vi "Multi-camera acquisition of images.vi"() -> ()   [LabVIEW 2018]
uses:
  LabViewDVPCamera/LabViewDVPCamera.lvlib
  <vilib>/picture/picture.llb/imagedata.ctl
panel:
  out "Capture frame rate 4":sgl
  out "Total frame rate 4":u32
  out "pFrameCount out 4":T1
  out "Capture frame rate 3":sgl
  out "Total frame rate 3":u32
  out "pFrameCount out 3":T1
  out "Capture frame rate 2":sgl
  out "Total frame rate 2":u32
  out "pFrameCount out 2":T1
  out "Capture frame rate":sgl
  out "Total frame rate":u32
  out "pFrameCount out":T1
  out "frame rate 4":dbl format="%#.5g"
  out "number 4":u64
  out "new picture 4":picture caption="新图片"
  in  "CloseFlg 4":i32
  in  "CameraList 4":u16(ring) caption="CameraList" items=["MGS130M-192.168.0.251"]
  out "Set 4":bool
  out "Open 4":bool
  out "Close 4":bool
  out "ScanCamera 4":bool
  out "handle 4":u32
  in  "image data 4":T2 caption="图像数据"
  out "Millisecond timing value 6":u32
  out "frame rate 3":dbl format="%#.5g"
  out "number 3":u64
  out "new picture 3":picture caption="新图片"
  in  "CloseFlg 3":i32
  in  "CameraList 3":u16(ring) caption="CameraList" items=["MGS130M-192.168.0.251"]
  in  "Set 3":bool
  in  "Open 3":bool
  in  "Close 3":bool
  in  "ScanCamera 3":bool
  out "handle 3":u32
  in  "image data 3":T2 caption="图像数据"
  out "Millisecond timing value 5":u32
  out "frame rate 2":dbl format="%#.5g"
  out "number 2":u64
  out "new picture 2":picture caption="新图片"
  out "CloseFlg 2":i32
  in  "CameraList 2":u16(ring) caption="CameraList" items=["MGS130M-192.168.0.251"]
  out "Set 2":bool
  out "Open 2":bool
  out "Close 2":bool
  out "ScanCamera 2":bool
  out "handle 2":u32
  in  "image data 2":T2 caption="图像数据"
  out "Millisecond timing value 4":u32
  in  "image data":T2 caption="图像数据"
  out "Millisecond timing value 3":u32
  out "frame rate":dbl format="%#.5g"
  out "number":u64
  out "new picture":picture caption="新图片"
  in  "CloseFlg":i32
  in  "CameraList":u16(ring) items=["MGS130M-192.168.0.251"]
  in  "Set":bool
  in  "Open":bool
  out "Close":bool
  in  "ScanCamera":bool
  out "handle":u32
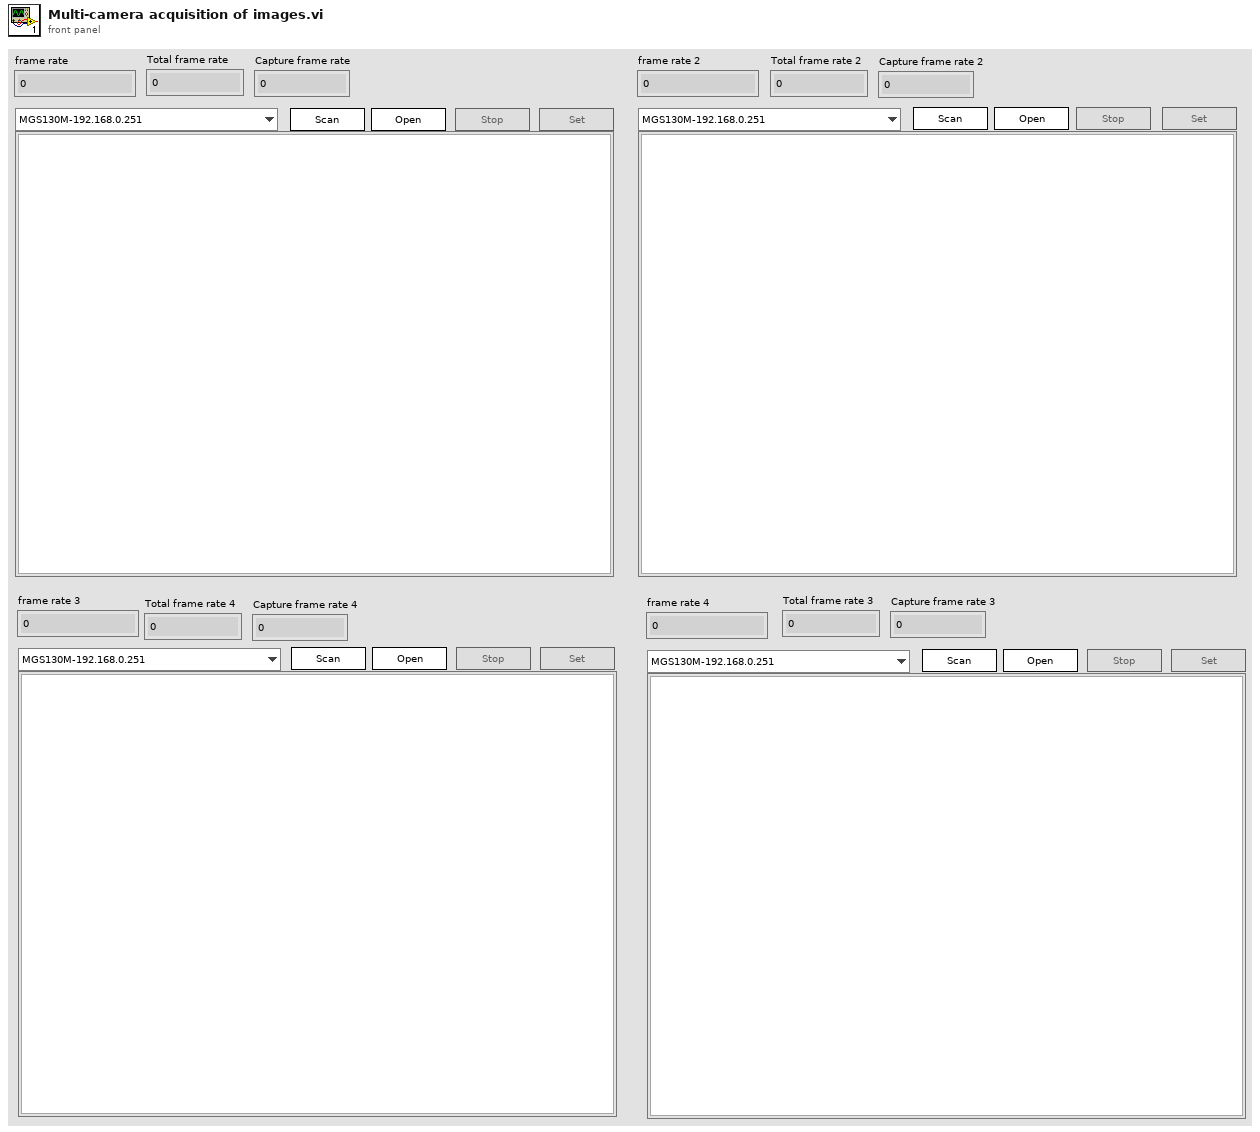
[diagram p1: front panel]
types:
  T1 = cluster{"uFrameCount":u32, "uFrameDrop":u32, "uFrameIgnore":u32, "uFrameError":u32, "uFrameOK":u32, "uFrameOut":u32, "uFrameResend":u32, "uFrameProc":u32, "fFrameRate":sgl, "fProcRate":sgl, "reserved[0]":i32, "reserved[1]":i32, "reserved[2]":i32, "reserved[3]":i32, "reserved[4]":i32, "reserved[5]":i32, "reserved[6]":i32, "reserved[7]":i32, "reserved[8]":i32, "reserved[9]":i32, "reserved[10]":i32, "reserved[11]":i32, "reserved[12]":i32, "reserved[13]":i32, "reserved[14]":i32, "reserved[15]":i32, "reserved[16]":i32, "reserved[17]":i32, "reserved[18]":i32, "reserved[19]":i32, "reserved[20]":i32, "reserved[21]":i32, "reserved[22]":i32, "reserved[23]":i32, "reserved[24]":i32, "reserved[25]":i32, "reserved[26]":i32, "reserved[27]":i32, "reserved[28]":i32, "reserved[29]":i32, "reserved[30]":i32, "reserved[31]":i32}
  T2 = typedef "imagedata.ctl" = cluster{"image type":i32, "image depth":i32, "image":u8[], "mask":u8[], "colors":u32[], "Rectangle":cluster{"left":i16, "top":i16, "right":i16, "bottom":i16}}
  T3 = enum8{"Enabled", "Disabled", "Disabled and Grayed Out"}
  T4 = typedef "LVStringsAndValuesArrayTypeDef_U16.ctl" = cluster{"String":string, "Value":u16}[]
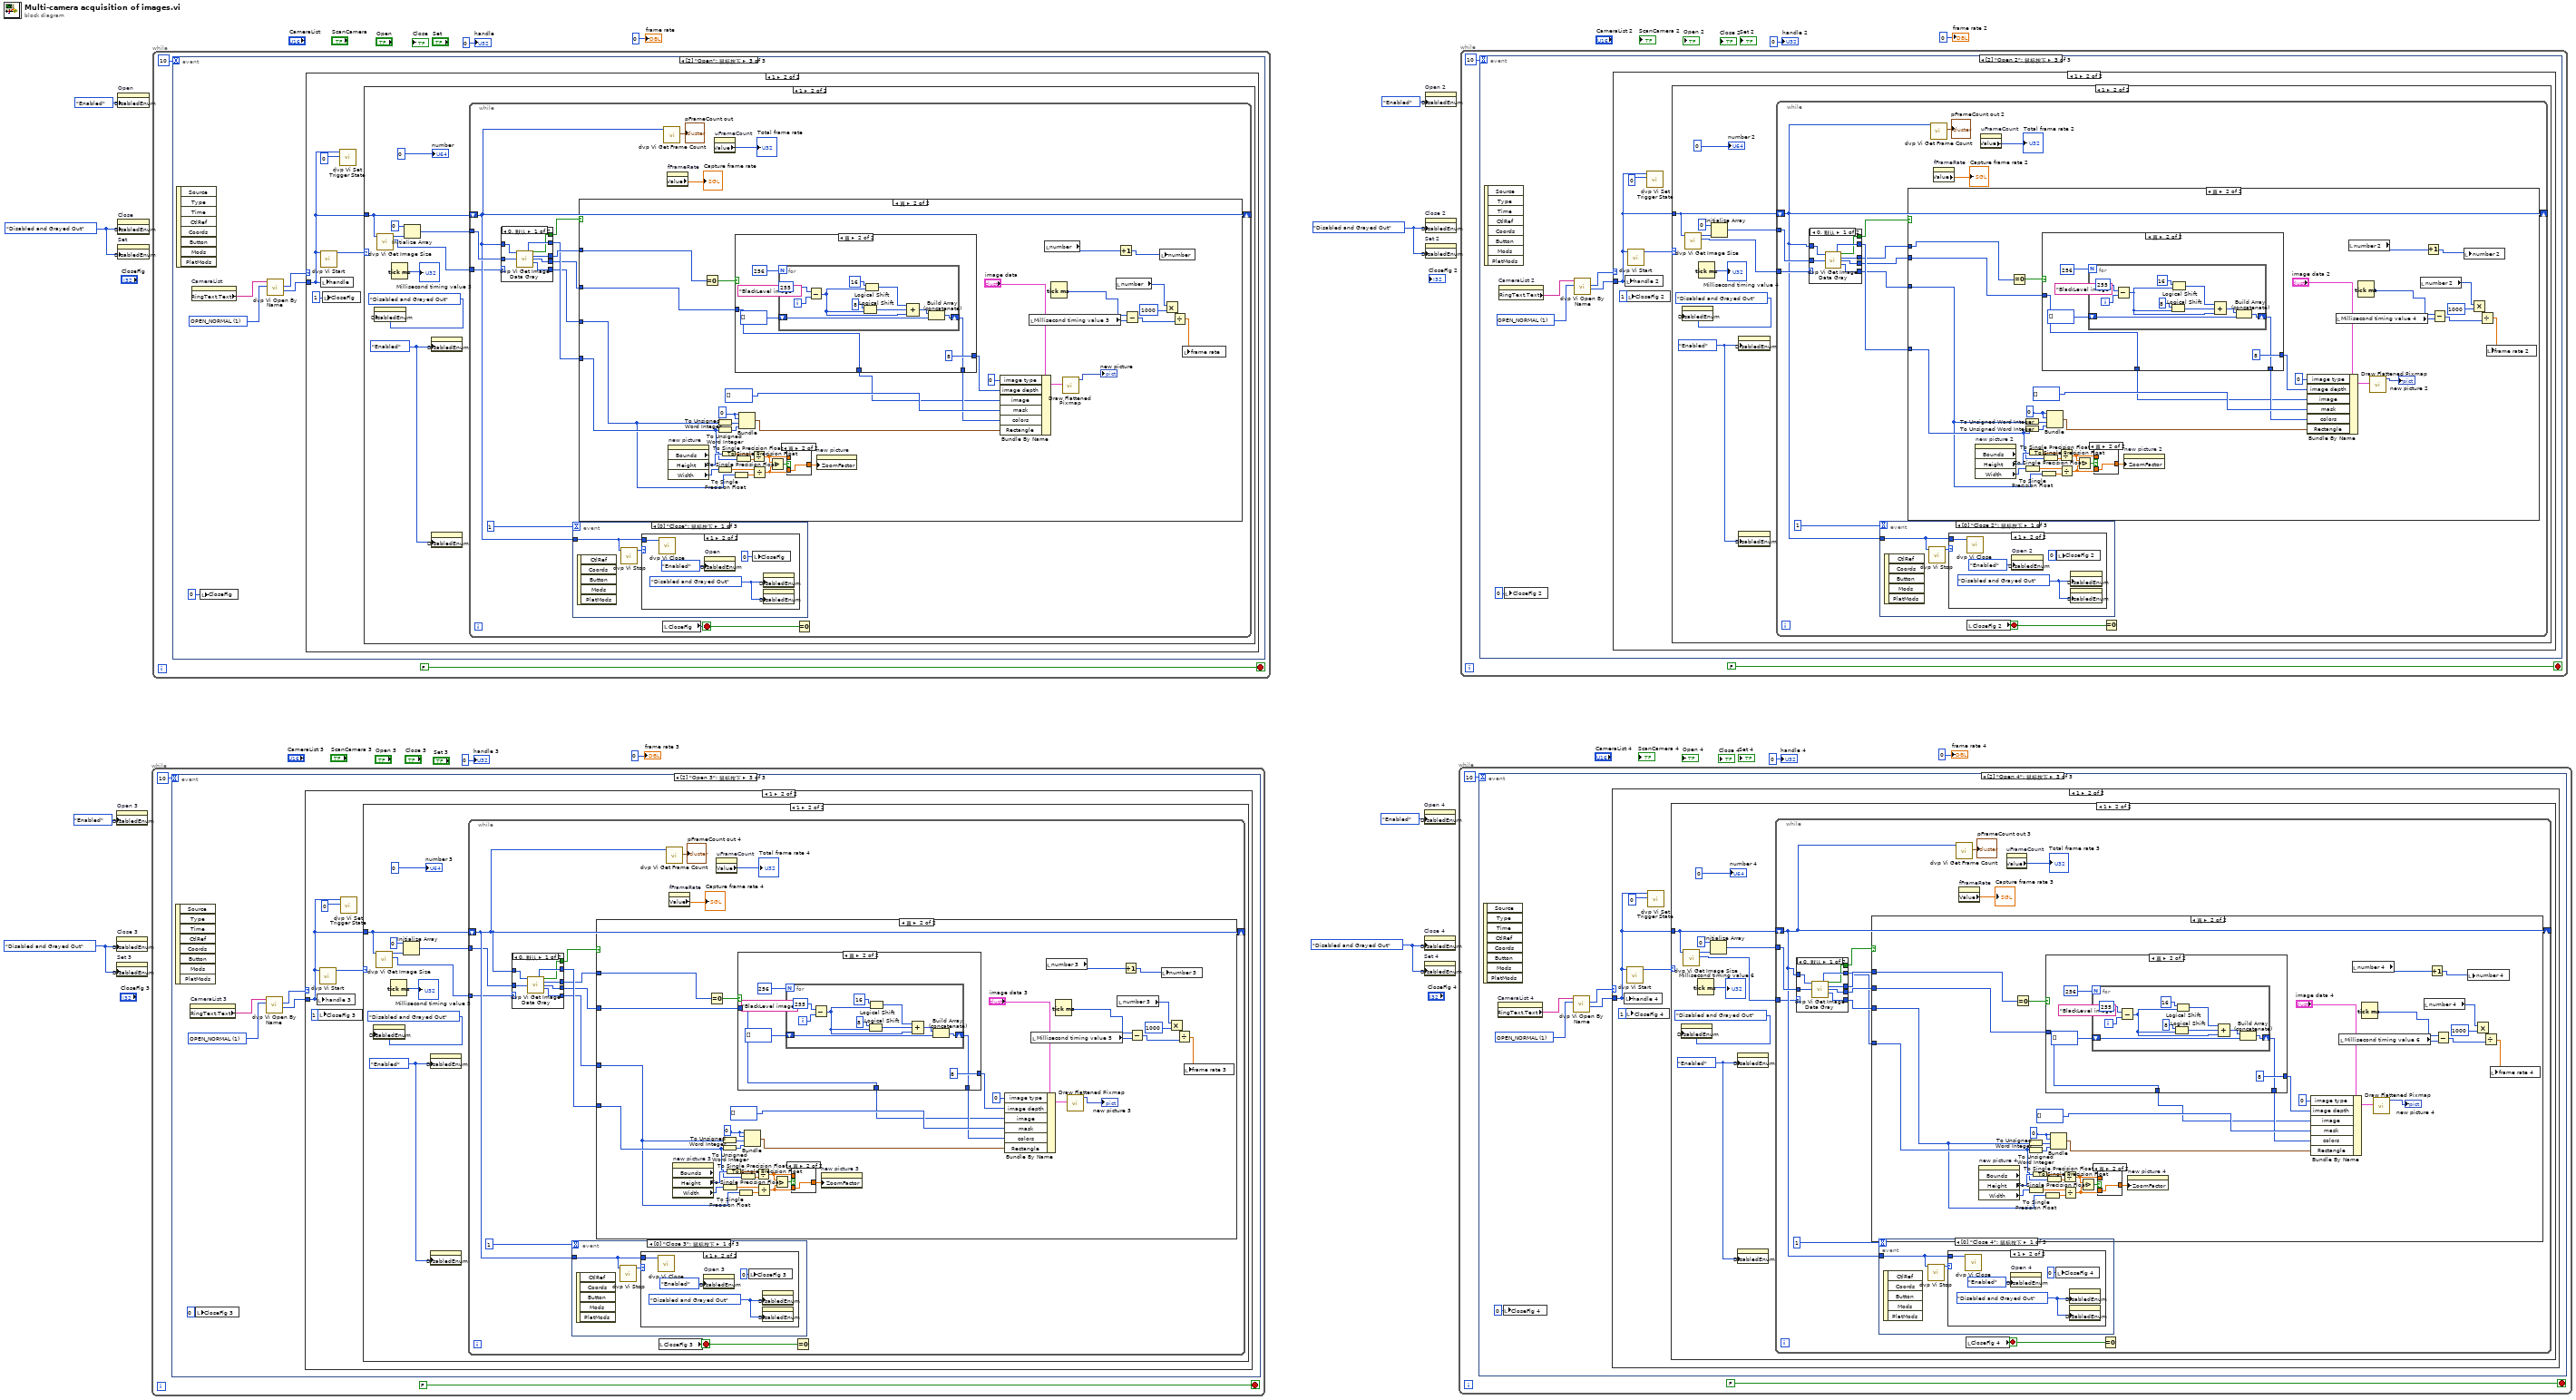
[diagram p0: block diagram]
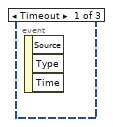
[diagram p2: hidden frame]
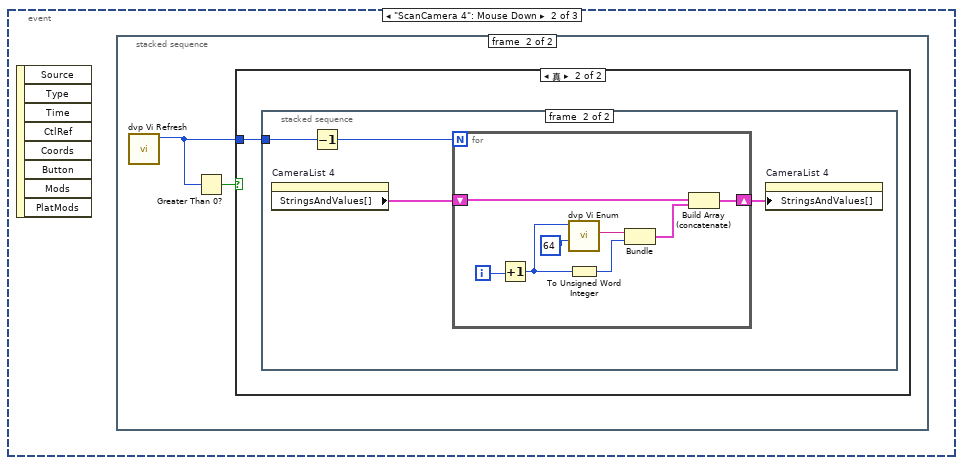
[diagram p3: hidden frame]
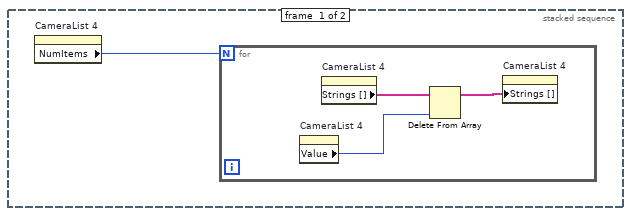
[diagram p4: hidden frame]
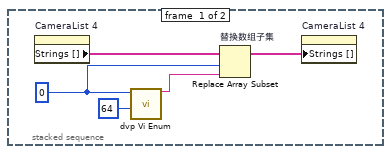
[diagram p6: hidden frame]
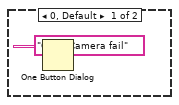
[diagram p7: hidden frame]
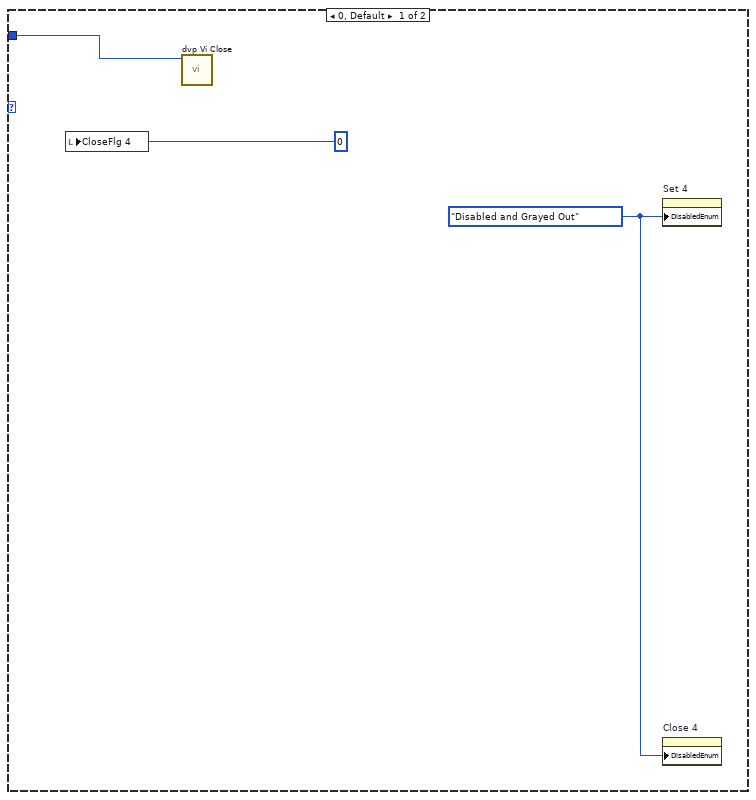
[diagram p8: hidden frame]
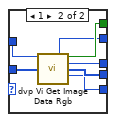
[diagram p9: hidden frame]
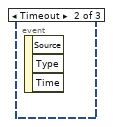
[diagram p11: hidden frame]
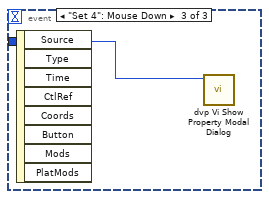
[diagram p12: hidden frame]
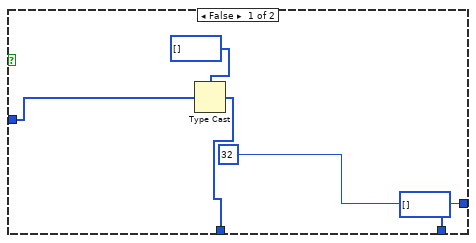
[diagram p15: hidden frame]
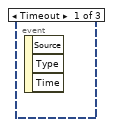
[diagram p16: hidden frame]
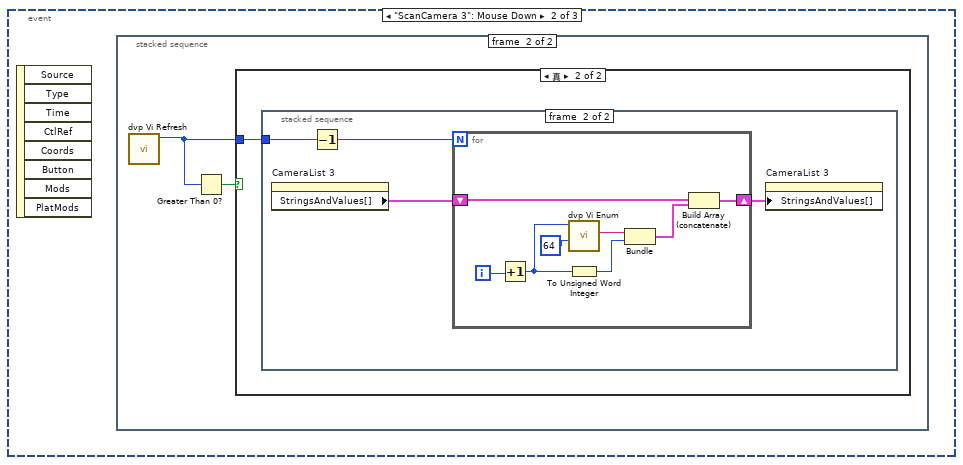
[diagram p17: hidden frame]
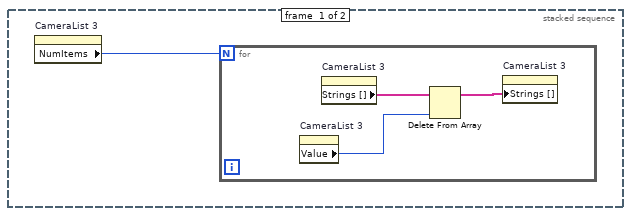
[diagram p18: hidden frame]
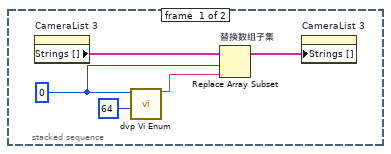
[diagram p20: hidden frame]
diagram:
  w3 = T3."Disabled and Grayed Out" ("禁用")
  w7 = T3."Disabled and Grayed Out" ("禁用")
  w11 = T3."Disabled and Grayed Out" ("禁用")
  w15 = T3."Disabled and Grayed Out" ("禁用")
  n1 = property on="Open 3" class="Bool"("DisabledEnum"=T3."Enabled" ("禁用")) -> ()  [unwired: 2 in, 2 out]
  n2 = property on="Close 3" class="Bool"("DisabledEnum"=w7) -> ()  [unwired: 2 in, 2 out]
  n3 = property on="Set 3" class="Bool"("DisabledEnum"=w7) -> ()  [unwired: 2 in, 2 out]
  n4 = property on="Open" class="Bool"("DisabledEnum"=T3."Enabled" ("禁用")) -> ()  [unwired: 2 in, 2 out]
  n5 = property on="Close" class="Bool"("DisabledEnum"=w15) -> ()  [unwired: 2 in, 2 out]
  n6 = property on="Set" class="Bool"("DisabledEnum"=w15) -> ()  [unwired: 2 in, 2 out]
  n7 = while {
    stop <- FALSE stop-if-true
    n8 = event shown="[2] \"Open 3\": 鼠标按下" {
      selector: _ -> [_ _ _]
      dyn-events: _ -> [_ _ _]
      timeout: 10 -> [_ _ _]
      event Timeout {
        n9 = event-data() -> ()  [unwired: 1 in, 3 out]
      }
      event "ScanCamera 3": Mouse Down {
        n10 = event-data() -> ()  [unwired: 1 in, 8 out]
        n11 = stacked-sequence "清除下拉列表的数据" {
          frame #0 {
            n12 = property on="CameraList 3" class="Ring (严格)"() -> ("NumItems"=w19:u32)  [unwired: 2 in, 2 out]
            n13 = for {
              N: w19 -> [_]
              n14 = property on="CameraList 3" class="Ring (严格)"() -> ("Value"=w21:u16)  [unwired: 2 in, 2 out]
              n15 = property on="CameraList 3" class="Ring (严格)"() -> ("Strings []"=w20:string[])  [unwired: 2 in, 2 out]
              n16 = Delete From Array ("删除数组元素")(array=w20, index=w21) -> (array with subset deleted=w22:string[])  [unwired: 1 in, 1 out]
              n17 = property on="CameraList 3" class="Ring (严格)"("Strings []"=w22) -> ()  [unwired: 2 in, 2 out]
            }
          }
          frame #1 {
            n18 = call "dvp Vi Refresh.vi"() -> ("pCount out"=w24:u32)  [unwired: 10 in, 1 out]
            n19 = Greater Than 0?(x=w24) -> (x > 0?=w23:bool)
            n20 = case shown="真" w23 {
              tunnel: w24 -> [_ w25]
              frame False {
              }
              frame True {
                n21 = stacked-sequence {
                  tunnel: w25 -> [_ w32]
                  frame #0 {
                    w26 = u32 0 ("index")
                    n22 = property on="CameraList 3" class="Ring (严格)"() -> ("Strings []"=w29:string[])  [unwired: 2 in, 2 out]
                    n23 = call "dvp Vi Enum.vi"("unSize"=u32 64, "index"=w26) -> ("friendlyName out"=w28:string)  [unwired: 8 in, 1 out]
                    n24 = Replace Array Subset "替换数组子集"(array=w29, new element=w28, index=w26) -> (w30:string[])
                    n25 = property on="CameraList 3" class="Ring (严格)"("Strings []"=w30) -> ()  [unwired: 2 in, 2 out]
                  }
                  frame #1 {
                    n26 = property on="CameraList 3" class="Ring (严格)"() -> ("StringsAndValues[]"=w34:T4)  [unwired: 2 in, 2 out]
                    n27 = Decrement(x=w32) -> (x-1=w31:u32)
                    n28 = for {
                      N: w31 -> [_]
                      shift-right: [w41] -> w33
                      shift-left: w34 -> [w39]
                      i -> [w36]
                      n29 = Increment(x=w36) -> (x+1=w35:i32)
                      n30 = call "dvp Vi Enum.vi"("unSize"=u32 64, "index"=w35) -> ("friendlyName out"=w42:string)  [unwired: 8 in, 1 out]
                      n31 = To Unsigned Word Integer(number=w35) -> (unsigned 16bit integer=w38:u16)
                      n32 = Bundle("friendlyName out"=w42, w38) -> (w40:cluster{"friendlyName out":string, u16})  [unwired: 1 in]
                      n33 = Build Array (concatenate)(w39, w40) -> (w41:T4)
                    }
                    n34 = property on="CameraList 3" class="Ring (严格)"("StringsAndValues[]"=w33) -> ()  [unwired: 2 in, 2 out]
                  }
                }
              }
            }
          }
        }
      }
      event "Open 3": Mouse Down {
        w45 = u32 1 items=["OPEN_OFFLINE", "OPEN_NORMAL"] ("type")
        n35 = event-data() -> ()  [unwired: 1 in, 8 out]
        n36 = property on="CameraList 3" class="Ring (严格)"() -> ("RingText.Text"=w44:string)  [unwired: 2 in, 2 out]
        n37 = local write "CloseFlg 3"(0 ("CloseFlg")) -> ()
        n38 = call "dvp Vi Open By Name.vi"("type"=w45, "friendlyName"=w44) -> ("pHandle out"=w47:u32, "function return"=w46:u32)  [unwired: 7 in, 1 out]
        n39 = case shown="1" w46 {
          tunnel: w47 -> [_ w49]
          frame 0, Default {
            n40 = One Button Dialog(message="Open Camera fail" ("消息")) -> ()  [unwired: 1 in, 1 out]
          }
          frame 1 {
            n41 = local write "handle 3"(w49) -> ()
            n42 = local write "CloseFlg 3"(1 ("CloseFlg")) -> ()
            n43 = call "dvp Vi Start.vi"("handle"=w49) -> ("function return"=w51:u32)  [unwired: 10 in]
            n44 = call "dvp Vi Set Trigger State.vi"("TriggerState"=0, "handle"=w49) -> ()  [unwired: 9 in, 1 out]
            n45 = case shown="1" w51 {
              tunnel: w49 -> [w55 w60]
              frame 0, Default {
                w54 = T3."Disabled and Grayed Out" ("禁用")
                n46 = local write "CloseFlg 3"(0 ("CloseFlg")) -> ()
                n47 = call "dvp Vi Close.vi"("handle"=w55) -> ()  [unwired: 10 in, 1 out]
                n48 = property on="Set 3" class="Bool"("DisabledEnum"=w54) -> ()  [unwired: 2 in, 2 out]
                n49 = property on="Close 3" class="Bool"("DisabledEnum"=w54) -> ()  [unwired: 2 in, 2 out]
              }
              frame 1 {
                w64 = T3."Enabled" ("禁用")
                n50 = property on="Open 3" class="Bool"("DisabledEnum"=T3."Disabled and Grayed Out" ("禁用")) -> ()  [unwired: 2 in, 2 out]
                n51 = call "dvp Vi Get Image Size.vi"("handle"=w60) -> ("pformat out"=w57:i32, "function return"=w59:u32)  [unwired: 9 in]
                n52 = Tick Count (ms)() -> (millisecond timer value=→"Millisecond timing value 5":u32)
                n53 = Initialize Array(u32 0 ("元素"), w59) -> (w61:u32[])
                n54 = property on="Set 3" class="Bool"("DisabledEnum"=w64) -> ()  [unwired: 2 in, 2 out]
                n55 = property on="Close 3" class="Bool"("DisabledEnum"=w64) -> ()  [unwired: 2 in, 2 out]
                n56 = while {
                  shift-right: [w72] -> _
                  shift-left: w60 -> [w72]
                  tunnel: w61 -> [w71]
                  tunnel: w57 -> [w70]
                  stop <- w77 stop-if-true
                  n57 = case shown="0, 默认" w70 {
                    tunnel: w71 -> [w85 w92]
                    tunnel: w72 -> [w84 w91]
                    tunnel: [w80 w90] -> w69
                    tunnel: [w82 w89] -> w66
                    tunnel: [w81 w88] -> w67
                    tunnel: [w83 w87] -> w68
                    tunnel: [w79 w86] -> w65
                    frame 0, Default {
                      n58 = call "dvp Vi Get Image Data Gray.vi"("handle"=w84, "pbuffer"=w85) -> ("piHeight out"=w83:i32, "function return"=w80:bool, "pformat out"=w81:i32, "pbuffer out"=w82:u8[], "piWidth out"=w79:i32)  [unwired: 9 in]
                    }
                    frame 1 {
                      n59 = call "dvp Vi Get Image Data Rgb.vi"("handle"=w91, "pbuffer"=w92) -> ("piHeight out"=w87:i32, "function return"=w90:bool, "pformat out"=w88:i32, "pbuffer out"=w89:u32[], "piWidth out"=w86:i32)  [unwired: 9 in]
                    }
                  }
                  n60 = event shown="[0] \"Close 3\": 鼠标按下" {
                    selector: _ -> [_ _ _]
                    dyn-events: _ -> [_ _ _]
                    timeout: 1 -> [_ _ _]
                    tunnel: w72 -> [w93 _ w99]
                    event "Close 3": Mouse Down {
                      n61 = event-data() -> ()  [unwired: 1 in, 5 out]
                      n62 = call "dvp Vi Stop.vi"("handle"=w93) -> ("function return"=w94:u32)  [unwired: 10 in]
                      n63 = case shown="1" w94 {
                        tunnel: w93 -> [_ w96]
                        frame 0, Default {
                        }
                        frame 1 {
                          w95 = T3."Disabled and Grayed Out" ("禁用")
                          n64 = call "dvp Vi Close.vi"("handle"=w96) -> ()  [unwired: 10 in, 1 out]
                          n65 = property on="Open 3" class="Bool"("DisabledEnum"=T3."Enabled" ("禁用")) -> ()  [unwired: 2 in, 2 out]
                          n66 = local write "CloseFlg 3"(0 ("CloseFlg")) -> ()
                          n67 = property on="Close 3" class="Bool"("DisabledEnum"=w95) -> ()  [unwired: 2 in, 2 out]
                          n68 = property on="Set 3" class="Bool"("DisabledEnum"=w95) -> ()  [unwired: 2 in, 2 out]
                        }
                      }
                    }
                    event Timeout {
                      n69 = event-data() -> ()  [unwired: 1 in, 3 out]
                    }
                    event "Set 3": Mouse Down {
                      n70 = event-data() -> ()  [unwired: 1 in, 8 out]
                      n71 = call "dvp Vi Show Property Modal Dialog.vi"("handle"=w99) -> ()  [unwired: 10 in, 1 out]
                    }
                  }
                  n72 = case shown="真" w69 {
                    tunnel: w66 -> [_ w102]
                    tunnel: w65 -> [_ w104]
                    tunnel: w68 -> [_ w105]
                    tunnel: w67 -> [_ w106]
                    frame False {
                    }
                    frame True {
                      w135 = u16 0
                      n73 = property on="new picture 3" class="Pict" props=["Bounds", "Height", "Width"]() -> ("Height"=w107:u32, "Width"=w108:u32)  [unwired: 2 in, 3 out]
                      n74 = Equal To 0?(x=w106) -> (x = 0?=w132:bool)
                      n75 = To Unsigned Word Integer(number=w104) -> (unsigned 16bit integer=w134:u16)
                      n76 = To Unsigned Word Integer(number=w105) -> (unsigned 16bit integer=w133:u16)
                      n77 = To Single Precision Float(number=w108) -> (single precision float=w115:sgl)
                      n78 = To Single Precision Float(number=w107) -> (single precision float=w109:sgl)
                      n79 = case shown="真" w132 {
                        tunnel: [32 u8 8 ("image depth")] -> w129
                        tunnel: [i32[] [] ("数组") w144] -> w127
                        tunnel: w102 -> [w139 w143]
                        tunnel: [w138 w143] -> w101
                        frame False {
                          n80 = Type Cast(type=u8[] [], x=w139) -> (*(type *) &x=w138:u8[])
                        }
                        frame True {
                          (unwired) "BlackLevel image"
                          n81 = for {
                            N: 256 -> [_]
                            shift-right: [w152] -> w144
                            shift-left: i32[] [] ("数组") -> [w151]
                            i -> [w148]
                            n82 = Subtract(x=255, y=w148) -> (x-y=w149:i32)
                            n83 = Logical Shift(y=i16 8, x=w149) -> (x << y=w154:i32)
                            n84 = Logical Shift(y=16 ("x"), x=w149) -> (x << y=w155:i32)
                            n85 = Compound Arithmetic op=ADD(w155, w154, w149) -> (w153:i32)
                            n86 = Build Array (concatenate)(w153, w151) -> (w152:i32[])
                          }
                        }
                      }
                      n87 = To Single Precision Float(number=w104) -> (single precision float=w111:sgl)
                      n88 = To Single Precision Float(number=w105) -> (single precision float=w110:sgl)
                      n89 = Bundle ("图像尺寸")(w135, w135, w134, w133) -> (w126:cluster{u16, u16, u16, u16})  [unwired: 1 in]
                      n90 = Divide(x=w109, y=w110) -> (x/y=w113:sgl)
                      n91 = Divide(x=w115, y=w111) -> (x/y=w114:sgl)
                      n92 = Greater?(x=w113, y=w114) -> (0:w112:bool)
                      n93 = case shown="真" w112 {
                        tunnel: w113 -> [w136 _]
                        tunnel: w114 -> [_ w137]
                        tunnel: [w136 w137] -> w116
                        frame False {
                        }
                        frame True {
                        }
                      }
                      n94 = property on="new picture 3" class="Pict"("ZoomFactor"=w116) -> ()  [unwired: 2 in, 2 out]
                      n95 = Bundle By Name(cluster="image data 3", "image type"=0, "image depth"=w129, "image"=w101, "mask"=u8[] [] ("无符号8位数组"), "colors"=w127, "Rectangle"=w126) -> (w130:T2)
                      n96 = local read "Millisecond timing value 5"() -> (w103:u32)
                      n97 = local read "number 3"() -> (w121:u64)
                      n98 = Tick Count (ms)() -> (millisecond timer value=w119:u32)
                      n99 = call <vilib>:"Draw Flattened Pixmap.vi"("image data"=w130) -> ("new picture"=→"new picture 3":picture)  [unwired: 8 in]
                      n100 = local read "number 3"() -> (w118:u64)
                      n101 = Increment(x=w121) -> (x+1=w120:u64)
                      n102 = Subtract(x=w119, y=w103) -> (x-y=w124:u32)
                      n103 = local write "number 3"(w120) -> ()
                      n104 = Multiply(x=w118, y=u64 1000) -> (x*y=w122:u64)
                      n105 = Divide(x=w122, y=w124) -> (x/y=w117:dbl)
                      n106 = local write "frame rate 3"(w117) -> ()
                    }
                  }
                  n107 = local read "CloseFlg 3"() -> (w76:i32)
                  n108 = call "dvp Vi Get Frame Count.vi"("handle"=w72) -> ("pFrameCount out"=→"pFrameCount out 4":T1)  [unwired: 9 in, 1 out]
                  n109 = property on="fFrameRate" class="DigNum (严格)"() -> ("Value"=→"Capture frame rate 4":sgl)  [unwired: 2 in, 2 out]
                  n110 = property on="uFrameCount" class="DigNum (严格)"() -> ("Value"=→"Total frame rate 4":u32)  [unwired: 2 in, 2 out]
                  n111 = Equal To 0?(x=w76) -> (x = 0?=w77:bool)
                }
                "number 3" <- u64 0
              }
            }
          }
        }
      }
    }
  }
  n112 = while {
    stop <- FALSE stop-if-true
    n113 = event shown="[2] \"Open\": 鼠标按下" {
      selector: _ -> [_ _ _]
      dyn-events: _ -> [_ _ _]
      timeout: 10 -> [_ _ _]
      event Timeout {
        n114 = event-data() -> ()  [unwired: 1 in, 3 out]
      }
      event "ScanCamera": Mouse Down {
        n115 = event-data() -> ()  [unwired: 1 in, 8 out]
        n116 = stacked-sequence "清除下拉列表的数据" {
          frame #0 {
            n117 = property on="CameraList" class="Ring (严格)"() -> ("NumItems"=w160:u32)  [unwired: 2 in, 2 out]
            n118 = for {
              N: w160 -> [_]
              n119 = property on="CameraList" class="Ring (严格)"() -> ("Value"=w162:u16)  [unwired: 2 in, 2 out]
              n120 = property on="CameraList" class="Ring (严格)"() -> ("Strings []"=w161:string[])  [unwired: 2 in, 2 out]
              n121 = Delete From Array ("删除数组元素")(array=w161, index=w162) -> (array with subset deleted=w163:string[])  [unwired: 1 in, 1 out]
              n122 = property on="CameraList" class="Ring (严格)"("Strings []"=w163) -> ()  [unwired: 2 in, 2 out]
            }
          }
          frame #1 {
            n123 = call "dvp Vi Refresh.vi"() -> ("pCount out"=w165:u32)  [unwired: 10 in, 1 out]
            n124 = Greater Than 0?(x=w165) -> (x > 0?=w164:bool)
            n125 = case shown="真" w164 {
              tunnel: w165 -> [_ w166]
              frame False {
              }
              frame True {
                n126 = stacked-sequence {
                  tunnel: w166 -> [_ w173]
                  frame #0 {
                    w167 = u32 0 ("index")
                    n127 = property on="CameraList" class="Ring (严格)"() -> ("Strings []"=w170:string[])  [unwired: 2 in, 2 out]
                    n128 = call "dvp Vi Enum.vi"("unSize"=u32 64, "index"=w167) -> ("friendlyName out"=w169:string)  [unwired: 8 in, 1 out]
                    n129 = Replace Array Subset "替换数组子集"(array=w170, new element=w169, index=w167) -> (w171:string[])
                    n130 = property on="CameraList" class="Ring (严格)"("Strings []"=w171) -> ()  [unwired: 2 in, 2 out]
                  }
                  frame #1 {
                    n131 = property on="CameraList" class="Ring (严格)"() -> ("StringsAndValues[]"=w175:T4)  [unwired: 2 in, 2 out]
                    n132 = Decrement(x=w173) -> (x-1=w172:u32)
                    n133 = for {
                      N: w172 -> [_]
                      shift-right: [w182] -> w174
                      shift-left: w175 -> [w180]
                      i -> [w177]
                      n134 = Increment(x=w177) -> (x+1=w176:i32)
                      n135 = call "dvp Vi Enum.vi"("unSize"=u32 64, "index"=w176) -> ("friendlyName out"=w183:string)  [unwired: 8 in, 1 out]
                      n136 = To Unsigned Word Integer(number=w176) -> (unsigned 16bit integer=w179:u16)
                      n137 = Bundle("friendlyName out"=w183, w179) -> (w181:cluster{"friendlyName out":string, u16})  [unwired: 1 in]
                      n138 = Build Array (concatenate)(w180, w181) -> (w182:T4)
                    }
                    n139 = property on="CameraList" class="Ring (严格)"("StringsAndValues[]"=w174) -> ()  [unwired: 2 in, 2 out]
                  }
                }
              }
            }
          }
        }
      }
      event "Open": Mouse Down {
        w186 = u32 1 items=["OPEN_OFFLINE", "OPEN_NORMAL"] ("type")
        n140 = event-data() -> ()  [unwired: 1 in, 8 out]
        n141 = property on="CameraList" class="Ring (严格)"() -> ("RingText.Text"=w185:string)  [unwired: 2 in, 2 out]
        n142 = local write "CloseFlg"(0 ("CloseFlg")) -> ()
        n143 = call "dvp Vi Open By Name.vi"("type"=w186, "friendlyName"=w185) -> ("pHandle out"=w188:u32, "function return"=w187:u32)  [unwired: 7 in, 1 out]
        n144 = case shown="1" w187 {
          tunnel: w188 -> [_ w190]
          frame 0, Default {
            n145 = One Button Dialog(message="Open Camera fail" ("消息")) -> ()  [unwired: 1 in, 1 out]
          }
          frame 1 {
            n146 = call "dvp Vi Start.vi"("handle"=w190) -> ("function return"=w192:u32)  [unwired: 10 in]
            n147 = local write "handle"(w190) -> ()
            n148 = local write "CloseFlg"(1 ("CloseFlg")) -> ()
            n149 = call "dvp Vi Set Trigger State.vi"("TriggerState"=0, "handle"=w190) -> ()  [unwired: 9 in, 1 out]
            n150 = case shown="1" w192 {
              tunnel: w190 -> [w196 w201]
              frame 0, Default {
                w195 = T3."Disabled and Grayed Out" ("禁用")
                n151 = local write "CloseFlg"(0 ("CloseFlg")) -> ()
                n152 = call "dvp Vi Close.vi"("handle"=w196) -> ()  [unwired: 10 in, 1 out]
                n153 = property on="Set" class="Bool"("DisabledEnum"=w195) -> ()  [unwired: 2 in, 2 out]
                n154 = property on="Close" class="Bool"("DisabledEnum"=w195) -> ()  [unwired: 2 in, 2 out]
              }
              frame 1 {
                w205 = T3."Enabled" ("禁用")
                n155 = property on="Open" class="Bool"("DisabledEnum"=T3."Disabled and Grayed Out" ("禁用")) -> ()  [unwired: 2 in, 2 out]
                n156 = call "dvp Vi Get Image Size.vi"("handle"=w201) -> ("pformat out"=w198:i32, "function return"=w200:u32)  [unwired: 9 in]
                n157 = Tick Count (ms)() -> (millisecond timer value=→"Millisecond timing value 3":u32)
                n158 = Initialize Array(u32 0 ("元素"), w200) -> (w202:u32[])
                n159 = property on="Set" class="Bool"("DisabledEnum"=w205) -> ()  [unwired: 2 in, 2 out]
                n160 = property on="Close" class="Bool"("DisabledEnum"=w205) -> ()  [unwired: 2 in, 2 out]
                n161 = while {
                  shift-right: [w207] -> _
                  shift-left: w201 -> [w207]
                  tunnel: w202 -> [w208]
                  tunnel: w198 -> [w206]
                  stop <- w218 stop-if-true
                  n162 = case shown="0, 默认" w206 {
                    tunnel: w208 -> [w226 w233]
                    tunnel: w207 -> [w225 w232]
                    tunnel: [w221 w231] -> w213
                    tunnel: [w223 w230] -> w209
                    tunnel: [w222 w229] -> w212
                    tunnel: [w224 w228] -> w211
                    tunnel: [w220 w227] -> w210
                    frame 0, Default {
                      n163 = call "dvp Vi Get Image Data Gray.vi"("handle"=w225, "pbuffer"=w226) -> ("piHeight out"=w224:i32, "function return"=w221:bool, "pformat out"=w222:i32, "pbuffer out"=w223:u8[], "piWidth out"=w220:i32)  [unwired: 9 in]
                    }
                    frame 1 {
                      n164 = call "dvp Vi Get Image Data Rgb.vi"("handle"=w232, "pbuffer"=w233) -> ("piHeight out"=w228:i32, "function return"=w231:bool, "pformat out"=w229:i32, "pbuffer out"=w230:u32[], "piWidth out"=w227:i32)  [unwired: 9 in]
                    }
                  }
                  n165 = event shown="[0] \"Close\": 鼠标按下" {
                    selector: _ -> [_ _ _]
                    dyn-events: _ -> [_ _ _]
                    timeout: 1 -> [_ _ _]
                    tunnel: w207 -> [w234 _ w240]
                    event "Close": Mouse Down {
                      n166 = event-data() -> ()  [unwired: 1 in, 5 out]
                      n167 = call "dvp Vi Stop.vi"("handle"=w234) -> ("function return"=w235:u32)  [unwired: 10 in]
                      n168 = case shown="1" w235 {
                        tunnel: w234 -> [_ w237]
                        frame 0, Default {
                        }
                        frame 1 {
                          w236 = T3."Disabled and Grayed Out" ("禁用")
                          n169 = call "dvp Vi Close.vi"("handle"=w237) -> ()  [unwired: 10 in, 1 out]
                          n170 = property on="Open" class="Bool"("DisabledEnum"=T3."Enabled" ("禁用")) -> ()  [unwired: 2 in, 2 out]
                          n171 = local write "CloseFlg"(0 ("CloseFlg")) -> ()
                          n172 = property on="Close" class="Bool"("DisabledEnum"=w236) -> ()  [unwired: 2 in, 2 out]
                          n173 = property on="Set" class="Bool"("DisabledEnum"=w236) -> ()  [unwired: 2 in, 2 out]
                        }
                      }
                    }
                    event Timeout {
                      n174 = event-data() -> ()  [unwired: 1 in, 3 out]
                    }
                    event "Set": Mouse Down {
                      n175 = event-data() -> ()  [unwired: 1 in, 8 out]
                      n176 = call "dvp Vi Show Property Modal Dialog.vi"("handle"=w240) -> ()  [unwired: 10 in, 1 out]
                    }
                  }
                  n177 = case shown="真" w213 {
                    tunnel: w209 -> [_ w243]
                    tunnel: w210 -> [_ w245]
                    tunnel: w211 -> [_ w246]
                    tunnel: w212 -> [_ w247]
                    frame False {
                    }
                    frame True {
                      w276 = u16 0
                      n178 = property on="new picture" class="Pict" props=["Bounds", "Height", "Width"]() -> ("Height"=w248:u32, "Width"=w249:u32)  [unwired: 2 in, 3 out]
                      n179 = Equal To 0?(x=w247) -> (x = 0?=w273:bool)
                      n180 = To Unsigned Word Integer(number=w245) -> (unsigned 16bit integer=w275:u16)
                      n181 = To Unsigned Word Integer(number=w246) -> (unsigned 16bit integer=w274:u16)
                      n182 = To Single Precision Float(number=w249) -> (single precision float=w256:sgl)
                      n183 = To Single Precision Float(number=w248) -> (single precision float=w250:sgl)
                      n184 = To Single Precision Float(number=w245) -> (single precision float=w252:sgl)
                      n185 = case shown="真" w273 {
                        tunnel: [32 u8 8 ("image depth")] -> w270
                        tunnel: [i32[] [] ("数组") w285] -> w268
                        tunnel: w243 -> [w280 w284]
                        tunnel: [w279 w284] -> w242
                        frame False {
                          n186 = Type Cast(type=u8[] [], x=w280) -> (*(type *) &x=w279:u8[])
                        }
                        frame True {
                          (unwired) "BlackLevel image"
                          n187 = for {
                            N: 256 -> [_]
                            shift-right: [w293] -> w285
                            shift-left: i32[] [] ("数组") -> [w292]
                            i -> [w289]
                            n188 = Subtract(x=255, y=w289) -> (x-y=w290:i32)
                            n189 = Logical Shift(y=i16 8, x=w290) -> (x << y=w295:i32)
                            n190 = Logical Shift(y=16 ("x"), x=w290) -> (x << y=w296:i32)
                            n191 = Compound Arithmetic op=ADD(w296, w295, w290) -> (w294:i32)
                            n192 = Build Array (concatenate)(w294, w292) -> (w293:i32[])
                          }
                        }
                      }
                      n193 = To Single Precision Float(number=w246) -> (single precision float=w251:sgl)
                      n194 = Bundle ("图像尺寸")(w276, w276, w275, w274) -> (w267:cluster{u16, u16, u16, u16})  [unwired: 1 in]
                      n195 = Divide(x=w250, y=w251) -> (x/y=w254:sgl)
                      n196 = Divide(x=w256, y=w252) -> (x/y=w255:sgl)
                      n197 = Greater?(x=w254, y=w255) -> (0:w253:bool)
                      n198 = case shown="真" w253 {
                        tunnel: w254 -> [w277 _]
                        tunnel: w255 -> [_ w278]
                        tunnel: [w277 w278] -> w257
                        frame False {
                        }
                        frame True {
                        }
                      }
                      n199 = property on="new picture" class="Pict"("ZoomFactor"=w257) -> ()  [unwired: 2 in, 2 out]
                      n200 = Bundle By Name(cluster="image data", "image type"=0, "image depth"=w270, "image"=w242, "mask"=u8[] [] ("无符号8位数组"), "colors"=w268, "Rectangle"=w267) -> (w271:T2)
                      n201 = local read "Millisecond timing value 3"() -> (w244:u32)
                      n202 = local read "number"() -> (w262:u64)
                      n203 = Tick Count (ms)() -> (millisecond timer value=w260:u32)
                      n204 = call <vilib>:"Draw Flattened Pixmap.vi"("image data"=w271) -> ("new picture"=→"new picture":picture)  [unwired: 8 in]
                      n205 = local read "number"() -> (w259:u64)
                      n206 = Increment(x=w262) -> (x+1=w261:u64)
                      n207 = Subtract(x=w260, y=w244) -> (x-y=w265:u32)
                      n208 = local write "number"(w261) -> ()
                      n209 = Multiply(x=w259, y=u64 1000) -> (x*y=w263:u64)
                      n210 = Divide(x=w263, y=w265) -> (x/y=w258:dbl)
                      n211 = local write "frame rate"(w258) -> ()
                    }
                  }
                  n212 = local read "CloseFlg"() -> (w217:i32)
                  n213 = call "dvp Vi Get Frame Count.vi"("handle"=w207) -> ("pFrameCount out"=→"pFrameCount out":T1)  [unwired: 9 in, 1 out]
                  n214 = property on="fFrameRate" class="DigNum (严格)"() -> ("Value"=→"Capture frame rate":sgl)  [unwired: 2 in, 2 out]
                  n215 = property on="uFrameCount" class="DigNum (严格)"() -> ("Value"=→"Total frame rate":u32)  [unwired: 2 in, 2 out]
                  n216 = Equal To 0?(x=w217) -> (x = 0?=w218:bool)
                }
                "number" <- u64 0
              }
            }
          }
        }
      }
    }
  }
  n217 = property on="Open 4" class="Bool"("DisabledEnum"=T3."Enabled" ("禁用")) -> ()  [unwired: 2 in, 2 out]
  n218 = property on="Close 4" class="Bool"("DisabledEnum"=w3) -> ()  [unwired: 2 in, 2 out]
  n219 = property on="Set 4" class="Bool"("DisabledEnum"=w3) -> ()  [unwired: 2 in, 2 out]
  n220 = property on="Open 2" class="Bool"("DisabledEnum"=T3."Enabled" ("禁用")) -> ()  [unwired: 2 in, 2 out]
  n221 = property on="Close 2" class="Bool"("DisabledEnum"=w11) -> ()  [unwired: 2 in, 2 out]
  n222 = property on="Set 2" class="Bool"("DisabledEnum"=w11) -> ()  [unwired: 2 in, 2 out]
  n223 = while {
    stop <- FALSE stop-if-true
    n224 = event shown="[2] \"Open 4\": 鼠标按下" {
      selector: _ -> [_ _ _]
      dyn-events: _ -> [_ _ _]
      timeout: 10 -> [_ _ _]
      event Timeout {
        n225 = event-data() -> ()  [unwired: 1 in, 3 out]
      }
      event "ScanCamera 4": Mouse Down {
        n226 = event-data() -> ()  [unwired: 1 in, 8 out]
        n227 = stacked-sequence "清除下拉列表的数据" {
          frame #0 {
            n228 = property on="CameraList 4" class="Ring (严格)"() -> ("NumItems"=w301:u32)  [unwired: 2 in, 2 out]
            n229 = for {
              N: w301 -> [_]
              n230 = property on="CameraList 4" class="Ring (严格)"() -> ("Value"=w303:u16)  [unwired: 2 in, 2 out]
              n231 = property on="CameraList 4" class="Ring (严格)"() -> ("Strings []"=w302:string[])  [unwired: 2 in, 2 out]
              n232 = Delete From Array ("删除数组元素")(array=w302, index=w303) -> (array with subset deleted=w304:string[])  [unwired: 1 in, 1 out]
              n233 = property on="CameraList 4" class="Ring (严格)"("Strings []"=w304) -> ()  [unwired: 2 in, 2 out]
            }
          }
          frame #1 {
            n234 = call "dvp Vi Refresh.vi"() -> ("pCount out"=w306:u32)  [unwired: 10 in, 1 out]
            n235 = Greater Than 0?(x=w306) -> (x > 0?=w305:bool)
            n236 = case shown="真" w305 {
              tunnel: w306 -> [_ w307]
              frame False {
              }
              frame True {
                n237 = stacked-sequence {
                  tunnel: w307 -> [_ w314]
                  frame #0 {
                    w308 = u32 0 ("index")
                    n238 = property on="CameraList 4" class="Ring (严格)"() -> ("Strings []"=w311:string[])  [unwired: 2 in, 2 out]
                    n239 = call "dvp Vi Enum.vi"("unSize"=u32 64, "index"=w308) -> ("friendlyName out"=w310:string)  [unwired: 8 in, 1 out]
                    n240 = Replace Array Subset "替换数组子集"(array=w311, new element=w310, index=w308) -> (w312:string[])
                    n241 = property on="CameraList 4" class="Ring (严格)"("Strings []"=w312) -> ()  [unwired: 2 in, 2 out]
                  }
                  frame #1 {
                    n242 = property on="CameraList 4" class="Ring (严格)"() -> ("StringsAndValues[]"=w316:T4)  [unwired: 2 in, 2 out]
                    n243 = Decrement(x=w314) -> (x-1=w313:u32)
                    n244 = for {
                      N: w313 -> [_]
                      shift-right: [w323] -> w315
                      shift-left: w316 -> [w321]
                      i -> [w318]
                      n245 = Increment(x=w318) -> (x+1=w317:i32)
                      n246 = call "dvp Vi Enum.vi"("unSize"=u32 64, "index"=w317) -> ("friendlyName out"=w324:string)  [unwired: 8 in, 1 out]
                      n247 = To Unsigned Word Integer(number=w317) -> (unsigned 16bit integer=w320:u16)
                      n248 = Bundle("friendlyName out"=w324, w320) -> (w322:cluster{"friendlyName out":string, u16})  [unwired: 1 in]
                      n249 = Build Array (concatenate)(w321, w322) -> (w323:T4)
                    }
                    n250 = property on="CameraList 4" class="Ring (严格)"("StringsAndValues[]"=w315) -> ()  [unwired: 2 in, 2 out]
                  }
                }
              }
            }
          }
        }
      }
      event "Open 4": Mouse Down {
        w327 = u32 1 items=["OPEN_OFFLINE", "OPEN_NORMAL"] ("type")
        n251 = event-data() -> ()  [unwired: 1 in, 8 out]
        n252 = property on="CameraList 4" class="Ring (严格)"() -> ("RingText.Text"=w326:string)  [unwired: 2 in, 2 out]
        n253 = local write "CloseFlg 4"(0 ("CloseFlg")) -> ()
        n254 = call "dvp Vi Open By Name.vi"("type"=w327, "friendlyName"=w326) -> ("pHandle out"=w329:u32, "function return"=w328:u32)  [unwired: 7 in, 1 out]
        n255 = case shown="1" w328 {
          tunnel: w329 -> [_ w331]
          frame 0, Default {
            n256 = One Button Dialog(message="Open Camera fail" ("消息")) -> ()  [unwired: 1 in, 1 out]
          }
          frame 1 {
            n257 = local write "handle 4"(w331) -> ()
            n258 = local write "CloseFlg 4"(1 ("CloseFlg")) -> ()
            n259 = call "dvp Vi Start.vi"("handle"=w331) -> ("function return"=w333:u32)  [unwired: 10 in]
            n260 = call "dvp Vi Set Trigger State.vi"("TriggerState"=0, "handle"=w331) -> ()  [unwired: 9 in, 1 out]
            n261 = case shown="1" w333 {
              tunnel: w331 -> [w337 w342]
              frame 0, Default {
                w336 = T3."Disabled and Grayed Out" ("禁用")
                n262 = local write "CloseFlg 4"(0 ("CloseFlg")) -> ()
                n263 = call "dvp Vi Close.vi"("handle"=w337) -> ()  [unwired: 10 in, 1 out]
                n264 = property on="Set 4" class="Bool"("DisabledEnum"=w336) -> ()  [unwired: 2 in, 2 out]
                n265 = property on="Close 4" class="Bool"("DisabledEnum"=w336) -> ()  [unwired: 2 in, 2 out]
              }
              frame 1 {
                w346 = T3."Enabled" ("禁用")
                n266 = property on="Open 4" class="Bool"("DisabledEnum"=T3."Disabled and Grayed Out" ("禁用")) -> ()  [unwired: 2 in, 2 out]
                n267 = call "dvp Vi Get Image Size.vi"("handle"=w342) -> ("pformat out"=w339:i32, "function return"=w341:u32)  [unwired: 9 in]
                n268 = Tick Count (ms)() -> (millisecond timer value=→"Millisecond timing value 6":u32)
                n269 = Initialize Array(u32 0 ("元素"), w341) -> (w343:u32[])
                n270 = property on="Set 4" class="Bool"("DisabledEnum"=w346) -> ()  [unwired: 2 in, 2 out]
                n271 = property on="Close 4" class="Bool"("DisabledEnum"=w346) -> ()  [unwired: 2 in, 2 out]
                n272 = while {
                  shift-right: [w353] -> _
                  shift-left: w342 -> [w353]
                  tunnel: w343 -> [w354]
                  tunnel: w339 -> [w352]
                  stop <- w359 stop-if-true
                  n273 = case shown="0, 默认" w352 {
                    tunnel: w354 -> [w367 w374]
                    tunnel: w353 -> [w366 w373]
                    tunnel: [w362 w372] -> w349
                    tunnel: [w364 w371] -> w351
                    tunnel: [w363 w370] -> w350
                    tunnel: [w365 w369] -> w347
                    tunnel: [w361 w368] -> w348
                    frame 0, Default {
                      n274 = call "dvp Vi Get Image Data Gray.vi"("handle"=w366, "pbuffer"=w367) -> ("piHeight out"=w365:i32, "function return"=w362:bool, "pformat out"=w363:i32, "pbuffer out"=w364:u8[], "piWidth out"=w361:i32)  [unwired: 9 in]
                    }
                    frame 1 {
                      n275 = call "dvp Vi Get Image Data Rgb.vi"("handle"=w373, "pbuffer"=w374) -> ("piHeight out"=w369:i32, "function return"=w372:bool, "pformat out"=w370:i32, "pbuffer out"=w371:u32[], "piWidth out"=w368:i32)  [unwired: 9 in]
                    }
                  }
                  n276 = case shown="真" w349 {
                    tunnel: w351 -> [_ w383]
                    tunnel: w348 -> [_ w386]
                    tunnel: w347 -> [_ w387]
                    tunnel: w350 -> [_ w388]
                    frame False {
                    }
                    frame True {
                      w417 = u16 0
                      n277 = property on="new picture 4" class="Pict" props=["Bounds", "Height", "Width"]() -> ("Height"=w389:u32, "Width"=w390:u32)  [unwired: 2 in, 3 out]
                      n278 = Equal To 0?(x=w388) -> (x = 0?=w414:bool)
                      n279 = To Unsigned Word Integer(number=w386) -> (unsigned 16bit integer=w416:u16)
                      n280 = To Unsigned Word Integer(number=w387) -> (unsigned 16bit integer=w415:u16)
                      n281 = To Single Precision Float(number=w390) -> (single precision float=w397:sgl)
                      n282 = To Single Precision Float(number=w389) -> (single precision float=w391:sgl)
                      n283 = To Single Precision Float(number=w386) -> (single precision float=w393:sgl)
                      n284 = case shown="真" w414 {
                        tunnel: [32 u8 8 ("image depth")] -> w411
                        tunnel: [i32[] [] ("数组") w426] -> w409
                        tunnel: [w421 w425] -> w384
                        tunnel: w383 -> [w420 w425]
                        frame False {
                          n285 = Type Cast(type=u8[] [], x=w420) -> (*(type *) &x=w421:u8[])
                        }
                        frame True {
                          (unwired) "BlackLevel image"
                          n286 = for {
                            N: 256 -> [_]
                            shift-right: [w434] -> w426
                            shift-left: i32[] [] ("数组") -> [w433]
                            i -> [w430]
                            n287 = Subtract(x=255, y=w430) -> (x-y=w431:i32)
                            n288 = Logical Shift(y=i16 8, x=w431) -> (x << y=w436:i32)
                            n289 = Logical Shift(y=16 ("x"), x=w431) -> (x << y=w437:i32)
                            n290 = Compound Arithmetic op=ADD(w437, w436, w431) -> (w435:i32)
                            n291 = Build Array (concatenate)(w435, w433) -> (w434:i32[])
                          }
                        }
                      }
                      n292 = To Single Precision Float(number=w387) -> (single precision float=w392:sgl)
                      n293 = Bundle ("图像尺寸")(w417, w417, w416, w415) -> (w408:cluster{u16, u16, u16, u16})  [unwired: 1 in]
                      n294 = Divide(x=w391, y=w392) -> (x/y=w395:sgl)
                      n295 = Divide(x=w397, y=w393) -> (x/y=w396:sgl)
                      n296 = Greater?(x=w395, y=w396) -> (0:w394:bool)
                      n297 = case shown="真" w394 {
                        tunnel: w395 -> [w418 _]
                        tunnel: w396 -> [_ w419]
                        tunnel: [w418 w419] -> w398
                        frame False {
                        }
                        frame True {
                        }
                      }
                      n298 = property on="new picture 4" class="Pict"("ZoomFactor"=w398) -> ()  [unwired: 2 in, 2 out]
                      n299 = Bundle By Name(cluster="image data 4", "image type"=0, "image depth"=w411, "image"=w384, "mask"=u8[] [] ("无符号8位数组"), "colors"=w409, "Rectangle"=w408) -> (w412:T2)
                      n300 = local read "Millisecond timing value 6"() -> (w385:u32)
                      n301 = local read "number 4"() -> (w403:u64)
                      n302 = Tick Count (ms)() -> (millisecond timer value=w401:u32)
                      n303 = call <vilib>:"Draw Flattened Pixmap.vi"("image data"=w412) -> ("new picture"=→"new picture 4":picture)  [unwired: 8 in]
                      n304 = local read "number 4"() -> (w400:u64)
                      n305 = Increment(x=w403) -> (x+1=w402:u64)
                      n306 = Subtract(x=w401, y=w385) -> (x-y=w406:u32)
                      n307 = local write "number 4"(w402) -> ()
                      n308 = Multiply(x=w400, y=u64 1000) -> (x*y=w404:u64)
                      n309 = Divide(x=w404, y=w406) -> (x/y=w399:dbl)
                      n310 = local write "frame rate 4"(w399) -> ()
                    }
                  }
                  n311 = event shown="[0] \"Close 4\": 鼠标按下" {
                    selector: _ -> [_ _ _]
                    dyn-events: _ -> [_ _ _]
                    timeout: 1 -> [_ _ _]
                    tunnel: w353 -> [w375 _ w381]
                    event "Close 4": Mouse Down {
                      n312 = event-data() -> ()  [unwired: 1 in, 5 out]
                      n313 = call "dvp Vi Stop.vi"("handle"=w375) -> ("function return"=w376:u32)  [unwired: 10 in]
                      n314 = case shown="1" w376 {
                        tunnel: w375 -> [_ w378]
                        frame 0, Default {
                        }
                        frame 1 {
                          w377 = T3."Disabled and Grayed Out" ("禁用")
                          n315 = call "dvp Vi Close.vi"("handle"=w378) -> ()  [unwired: 10 in, 1 out]
                          n316 = property on="Open 4" class="Bool"("DisabledEnum"=T3."Enabled" ("禁用")) -> ()  [unwired: 2 in, 2 out]
                          n317 = local write "CloseFlg 4"(0 ("CloseFlg")) -> ()
                          n318 = property on="Close 4" class="Bool"("DisabledEnum"=w377) -> ()  [unwired: 2 in, 2 out]
                          n319 = property on="Set 4" class="Bool"("DisabledEnum"=w377) -> ()  [unwired: 2 in, 2 out]
                        }
                      }
                    }
                    event Timeout {
                      n320 = event-data() -> ()  [unwired: 1 in, 3 out]
                    }
                    event "Set 4": Mouse Down {
                      n321 = event-data() -> ()  [unwired: 1 in, 8 out]
                      n322 = call "dvp Vi Show Property Modal Dialog.vi"("handle"=w381) -> ()  [unwired: 10 in, 1 out]
                    }
                  }
                  n323 = call "dvp Vi Get Frame Count.vi"("handle"=w353) -> ("pFrameCount out"=→"pFrameCount out 3":T1)  [unwired: 9 in, 1 out]
                  n324 = property on="fFrameRate" class="DigNum (严格)"() -> ("Value"=→"Capture frame rate 3":sgl)  [unwired: 2 in, 2 out]
                  n325 = local read "CloseFlg 4"() -> (w358:i32)
                  n326 = property on="uFrameCount" class="DigNum (严格)"() -> ("Value"=→"Total frame rate 3":u32)  [unwired: 2 in, 2 out]
                  n327 = Equal To 0?(x=w358) -> (x = 0?=w359:bool)
                }
                "number 4" <- u64 0
              }
            }
          }
        }
      }
    }
  }
  n328 = while {
    stop <- FALSE stop-if-true
    n329 = event shown="[2] \"Open 2\": 鼠标按下" {
      selector: _ -> [_ _ _]
      dyn-events: _ -> [_ _ _]
      timeout: 10 -> [_ _ _]
      event Timeout {
        n330 = event-data() -> ()  [unwired: 1 in, 3 out]
      }
      event "ScanCamera 2": Mouse Down {
        n331 = event-data() -> ()  [unwired: 1 in, 8 out]
        n332 = stacked-sequence "清除下拉列表的数据" {
          frame #0 {
            n333 = property on="CameraList 2" class="Ring (严格)"() -> ("NumItems"=w442:u32)  [unwired: 2 in, 2 out]
            n334 = for {
              N: w442 -> [_]
              n335 = property on="CameraList 2" class="Ring (严格)"() -> ("Value"=w444:u16)  [unwired: 2 in, 2 out]
              n336 = property on="CameraList 2" class="Ring (严格)"() -> ("Strings []"=w443:string[])  [unwired: 2 in, 2 out]
              n337 = Delete From Array ("删除数组元素")(array=w443, index=w444) -> (array with subset deleted=w445:string[])  [unwired: 1 in, 1 out]
              n338 = property on="CameraList 2" class="Ring (严格)"("Strings []"=w445) -> ()  [unwired: 2 in, 2 out]
            }
          }
          frame #1 {
            n339 = call "dvp Vi Refresh.vi"() -> ("pCount out"=w447:u32)  [unwired: 10 in, 1 out]
            n340 = Greater Than 0?(x=w447) -> (x > 0?=w446:bool)
            n341 = case shown="真" w446 {
              tunnel: w447 -> [_ w448]
              frame False {
              }
              frame True {
                n342 = stacked-sequence {
                  tunnel: w448 -> [_ w455]
                  frame #0 {
                    w449 = u32 0 ("index")
                    n343 = property on="CameraList 2" class="Ring (严格)"() -> ("Strings []"=w452:string[])  [unwired: 2 in, 2 out]
                    n344 = call "dvp Vi Enum.vi"("unSize"=u32 64, "index"=w449) -> ("friendlyName out"=w451:string)  [unwired: 8 in, 1 out]
                    n345 = Replace Array Subset "替换数组子集"(array=w452, new element=w451, index=w449) -> (w453:string[])
                    n346 = property on="CameraList 2" class="Ring (严格)"("Strings []"=w453) -> ()  [unwired: 2 in, 2 out]
                  }
                  frame #1 {
                    n347 = property on="CameraList 2" class="Ring (严格)"() -> ("StringsAndValues[]"=w457:T4)  [unwired: 2 in, 2 out]
                    n348 = Decrement(x=w455) -> (x-1=w454:u32)
                    n349 = for {
                      N: w454 -> [_]
                      shift-right: [w464] -> w456
                      shift-left: w457 -> [w462]
                      i -> [w459]
                      n350 = Increment(x=w459) -> (x+1=w458:i32)
                      n351 = call "dvp Vi Enum.vi"("unSize"=u32 64, "index"=w458) -> ("friendlyName out"=w465:string)  [unwired: 8 in, 1 out]
                      n352 = To Unsigned Word Integer(number=w458) -> (unsigned 16bit integer=w461:u16)
                      n353 = Bundle("friendlyName out"=w465, w461) -> (w463:cluster{"friendlyName out":string, u16})  [unwired: 1 in]
                      n354 = Build Array (concatenate)(w462, w463) -> (w464:T4)
                    }
                    n355 = property on="CameraList 2" class="Ring (严格)"("StringsAndValues[]"=w456) -> ()  [unwired: 2 in, 2 out]
                  }
                }
              }
            }
          }
        }
      }
      event "Open 2": Mouse Down {
        w468 = u32 1 items=["OPEN_OFFLINE", "OPEN_NORMAL"] ("type")
        n356 = event-data() -> ()  [unwired: 1 in, 8 out]
        n357 = property on="CameraList 2" class="Ring (严格)"() -> ("RingText.Text"=w467:string)  [unwired: 2 in, 2 out]
        n358 = local write "CloseFlg 2"(0 ("CloseFlg")) -> ()
        n359 = call "dvp Vi Open By Name.vi"("type"=w468, "friendlyName"=w467) -> ("pHandle out"=w470:u32, "function return"=w469:u32)  [unwired: 7 in, 1 out]
        n360 = case shown="1" w469 {
          tunnel: w470 -> [_ w472]
          frame 0, Default {
            n361 = One Button Dialog(message="Open Camera fail" ("消息")) -> ()  [unwired: 1 in, 1 out]
          }
          frame 1 {
            n362 = local write "handle 2"(w472) -> ()
            n363 = local write "CloseFlg 2"(1 ("CloseFlg")) -> ()
            n364 = call "dvp Vi Start.vi"("handle"=w472) -> ("function return"=w474:u32)  [unwired: 10 in]
            n365 = call "dvp Vi Set Trigger State.vi"("TriggerState"=0, "handle"=w472) -> ()  [unwired: 9 in, 1 out]
            n366 = case shown="1" w474 {
              tunnel: w472 -> [w478 w483]
              frame 0, Default {
                w477 = T3."Disabled and Grayed Out" ("禁用")
                n367 = local write "CloseFlg 2"(0 ("CloseFlg")) -> ()
                n368 = call "dvp Vi Close.vi"("handle"=w478) -> ()  [unwired: 10 in, 1 out]
                n369 = property on="Set 2" class="Bool"("DisabledEnum"=w477) -> ()  [unwired: 2 in, 2 out]
                n370 = property on="Close 2" class="Bool"("DisabledEnum"=w477) -> ()  [unwired: 2 in, 2 out]
              }
              frame 1 {
                w487 = T3."Enabled" ("禁用")
                n371 = property on="Open 2" class="Bool"("DisabledEnum"=T3."Disabled and Grayed Out" ("禁用")) -> ()  [unwired: 2 in, 2 out]
                n372 = call "dvp Vi Get Image Size.vi"("handle"=w483) -> ("pformat out"=w480:i32, "function return"=w482:u32)  [unwired: 9 in]
                n373 = Tick Count (ms)() -> (millisecond timer value=→"Millisecond timing value 4":u32)
                n374 = Initialize Array(u32 0 ("元素"), w482) -> (w484:u32[])
                n375 = property on="Set 2" class="Bool"("DisabledEnum"=w487) -> ()  [unwired: 2 in, 2 out]
                n376 = property on="Close 2" class="Bool"("DisabledEnum"=w487) -> ()  [unwired: 2 in, 2 out]
                n377 = while {
                  shift-right: [w488] -> _
                  shift-left: w483 -> [w488]
                  tunnel: w484 -> [w489]
                  tunnel: w480 -> [w495]
                  stop <- w500 stop-if-true
                  n378 = case shown="0, 默认" w495 {
                    tunnel: w489 -> [w508 w515]
                    tunnel: w488 -> [w507 w514]
                    tunnel: [w503 w513] -> w494
                    tunnel: [w505 w512] -> w491
                    tunnel: [w504 w511] -> w492
                    tunnel: [w506 w510] -> w493
                    tunnel: [w502 w509] -> w490
                    frame 0, Default {
                      n379 = call "dvp Vi Get Image Data Gray.vi"("handle"=w507, "pbuffer"=w508) -> ("piHeight out"=w506:i32, "function return"=w503:bool, "pformat out"=w504:i32, "pbuffer out"=w505:u8[], "piWidth out"=w502:i32)  [unwired: 9 in]
                    }
                    frame 1 {
                      n380 = call "dvp Vi Get Image Data Rgb.vi"("handle"=w514, "pbuffer"=w515) -> ("piHeight out"=w510:i32, "function return"=w513:bool, "pformat out"=w511:i32, "pbuffer out"=w512:u32[], "piWidth out"=w509:i32)  [unwired: 9 in]
                    }
                  }
                  n381 = event shown="[0] \"Close 2\": 鼠标按下" {
                    selector: _ -> [_ _ _]
                    dyn-events: _ -> [_ _ _]
                    timeout: 1 -> [_ _ _]
                    tunnel: w488 -> [w516 _ w522]
                    event "Close 2": Mouse Down {
                      n382 = event-data() -> ()  [unwired: 1 in, 5 out]
                      n383 = call "dvp Vi Stop.vi"("handle"=w516) -> ("function return"=w517:u32)  [unwired: 10 in]
                      n384 = case shown="1" w517 {
                        tunnel: w516 -> [_ w519]
                        frame 0, Default {
                        }
                        frame 1 {
                          w518 = T3."Disabled and Grayed Out" ("禁用")
                          n385 = call "dvp Vi Close.vi"("handle"=w519) -> ()  [unwired: 10 in, 1 out]
                          n386 = property on="Open 2" class="Bool"("DisabledEnum"=T3."Enabled" ("禁用")) -> ()  [unwired: 2 in, 2 out]
                          n387 = local write "CloseFlg 2"(0 ("CloseFlg")) -> ()
                          n388 = property on="Close 2" class="Bool"("DisabledEnum"=w518) -> ()  [unwired: 2 in, 2 out]
                          n389 = property on="Set 2" class="Bool"("DisabledEnum"=w518) -> ()  [unwired: 2 in, 2 out]
                        }
                      }
                    }
                    event Timeout {
                      n390 = event-data() -> ()  [unwired: 1 in, 3 out]
                    }
                    event "Set 2": Mouse Down {
                      n391 = event-data() -> ()  [unwired: 1 in, 8 out]
                      n392 = call "dvp Vi Show Property Modal Dialog.vi"("handle"=w522) -> ()  [unwired: 10 in, 1 out]
                    }
                  }
                  n393 = case shown="真" w494 {
                    tunnel: w491 -> [_ w525]
                    tunnel: w490 -> [_ w528]
                    tunnel: w493 -> [_ w529]
                    tunnel: w492 -> [_ w526]
                    frame False {
                    }
                    frame True {
                      w558 = u16 0
                      n394 = property on="new picture 2" class="Pict" props=["Bounds", "Height", "Width"]() -> ("Height"=w530:u32, "Width"=w531:u32)  [unwired: 2 in, 3 out]
                      n395 = Equal To 0?(x=w526) -> (x = 0?=w555:bool)
                      n396 = To Unsigned Word Integer(number=w528) -> (unsigned 16bit integer=w557:u16)
                      n397 = To Unsigned Word Integer(number=w529) -> (unsigned 16bit integer=w556:u16)
                      n398 = To Single Precision Float(number=w531) -> (single precision float=w538:sgl)
                      n399 = To Single Precision Float(number=w530) -> (single precision float=w532:sgl)
                      n400 = To Single Precision Float(number=w528) -> (single precision float=w534:sgl)
                      n401 = case shown="真" w555 {
                        tunnel: [32 u8 8 ("image depth")] -> w552
                        tunnel: [i32[] [] ("数组") w567] -> w550
                        tunnel: w525 -> [w562 w566]
                        tunnel: [w561 w566] -> w524
                        frame False {
                          n402 = Type Cast(type=u8[] [], x=w562) -> (*(type *) &x=w561:u8[])
                        }
                        frame True {
                          (unwired) "BlackLevel image"
                          n403 = for {
                            N: 256 -> [_]
                            shift-right: [w575] -> w567
                            shift-left: i32[] [] ("数组") -> [w574]
                            i -> [w571]
                            n404 = Subtract(x=255, y=w571) -> (x-y=w572:i32)
                            n405 = Logical Shift(y=i16 8, x=w572) -> (x << y=w577:i32)
                            n406 = Logical Shift(y=16 ("x"), x=w572) -> (x << y=w578:i32)
                            n407 = Compound Arithmetic op=ADD(w578, w577, w572) -> (w576:i32)
                            n408 = Build Array (concatenate)(w576, w574) -> (w575:i32[])
                          }
                        }
                      }
                      n409 = To Single Precision Float(number=w529) -> (single precision float=w533:sgl)
                      n410 = Bundle ("图像尺寸")(w558, w558, w557, w556) -> (w549:cluster{u16, u16, u16, u16})  [unwired: 1 in]
                      n411 = Divide(x=w532, y=w533) -> (x/y=w536:sgl)
                      n412 = Divide(x=w538, y=w534) -> (x/y=w537:sgl)
                      n413 = Greater?(x=w536, y=w537) -> (0:w535:bool)
                      n414 = case shown="真" w535 {
                        tunnel: w536 -> [w559 _]
                        tunnel: w537 -> [_ w560]
                        tunnel: [w559 w560] -> w539
                        frame False {
                        }
                        frame True {
                        }
                      }
                      n415 = property on="new picture 2" class="Pict"("ZoomFactor"=w539) -> ()  [unwired: 2 in, 2 out]
                      n416 = Bundle By Name(cluster="image data 2", "image type"=0, "image depth"=w552, "image"=w524, "mask"=u8[] [] ("无符号8位数组"), "colors"=w550, "Rectangle"=w549) -> (w553:T2)
                      n417 = local read "Millisecond timing value 4"() -> (w527:u32)
                      n418 = local read "number 2"() -> (w544:u64)
                      n419 = Tick Count (ms)() -> (millisecond timer value=w542:u32)
                      n420 = call <vilib>:"Draw Flattened Pixmap.vi"("image data"=w553) -> ("new picture"=→"new picture 2":picture)  [unwired: 8 in]
                      n421 = local read "number 2"() -> (w541:u64)
                      n422 = Increment(x=w544) -> (x+1=w543:u64)
                      n423 = Subtract(x=w542, y=w527) -> (x-y=w547:u32)
                      n424 = local write "number 2"(w543) -> ()
                      n425 = Multiply(x=w541, y=u64 1000) -> (x*y=w545:u64)
                      n426 = Divide(x=w545, y=w547) -> (x/y=w540:dbl)
                      n427 = local write "frame rate 2"(w540) -> ()
                    }
                  }
                  n428 = call "dvp Vi Get Frame Count.vi"("handle"=w488) -> ("pFrameCount out"=→"pFrameCount out 2":T1)  [unwired: 9 in, 1 out]
                  n429 = property on="fFrameRate" class="DigNum (严格)"() -> ("Value"=→"Capture frame rate 2":sgl)  [unwired: 2 in, 2 out]
                  n430 = local read "CloseFlg 2"() -> (w499:i32)
                  n431 = property on="uFrameCount" class="DigNum (严格)"() -> ("Value"=→"Total frame rate 2":u32)  [unwired: 2 in, 2 out]
                  n432 = Equal To 0?(x=w499) -> (x = 0?=w500:bool)
                }
                "number 2" <- u64 0
              }
            }
          }
        }
      }
    }
  }
  "handle" <- u32 0 ("handle")
  "frame rate" <- 0
  "handle 2" <- u32 0 ("handle")
  "frame rate 2" <- 0
  "handle 3" <- u32 0 ("handle")
  "frame rate 3" <- 0
  "handle 4" <- u32 0 ("handle")
  "frame rate 4" <- 0
